vi "TS530 set power.vi"(1 "error in":errorcluster, 2 "Power Range":T1(ring), 3 "Power Bias":enum16{"0%", "20%", "40%", "60%", "80%", "100%"}(ring), 4 "GPIB Address":refnum<visa-resource-name>) -> (0 "error out":errorcluster={"status"=TRUE, "code"=2, "source"="GPIB Write in \rUntitled 1"})   [LabVIEW 2021]
panel:
  # "TS530 Set Power"
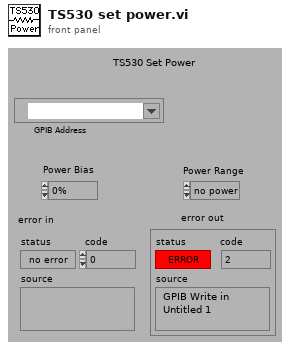
[diagram p1: front panel]
types:
  T1 = enum16{"no power", "1uW", "10uW", "100uW", "1mW", "10mW", "100mW", "1W"}
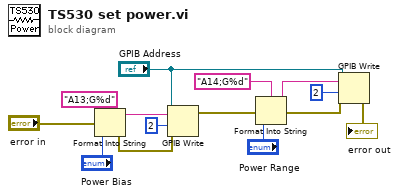
[diagram p0: block diagram]
diagram:
  n1 = Format Into String(format string="A13;G%d", error in="error in", "Power Bias") -> (resulting string=w7:string, error out=w5:errorcluster)  [unwired: 1 in]
  n2 = GPIB Write(0:"GPIB Address", 1:w7, 2:2, 3:w5) -> (6:w2:errorcluster)  [unwired: 1 in, 1 out]
  n3 = Format Into String(format string="A14;G%d", error in=w2, "Power Range") -> (resulting string=w12:string, error out=w4:errorcluster)  [unwired: 1 in]
  n4 = GPIB Write(0:"GPIB Address", 1:w12, 2:2, 3:w4) -> (6:→"error out":errorcluster)  [unwired: 1 in, 1 out]
